vi "OSF Template.vi"(8 "error in":errorcluster, 9 "Proposal Data":T1, 10 "Token":string, 11 "OSF API URL":string="https://api.osf.io/v2/") -> (0 "error out":errorcluster)   [LabVIEW 2020]
uses:
  Utilities/iCalendar/Extract iCalendar String.ctl
  <vilib>/httpClient/LabVIEWHTTPClient.lvlib
  <vilib>/JDP Science/JSONtext/JSONtext.lvlib
panel:
  in  "Path to item":string="home1"
  in  "content":string
  in  "ID":string
  out "Display Text 2":string
  out "Display Text":string
  in  "Act":bool=TRUE
  in  "Responce body":string
  in  "Parse from":enum16{"Proposal HTML:", "Proposal cluster"}(ring)=enum."Proposal cluster"
  out "reply":string
  out "headers":string
  in  "Proposal document":path=path "C:/Users/l121767/Dropbox/Projects/FAIR/Project files/Proposal/National High Magnetic Field Laboratory - Users Program.html"
  out "resulting string":string
  out "body":string
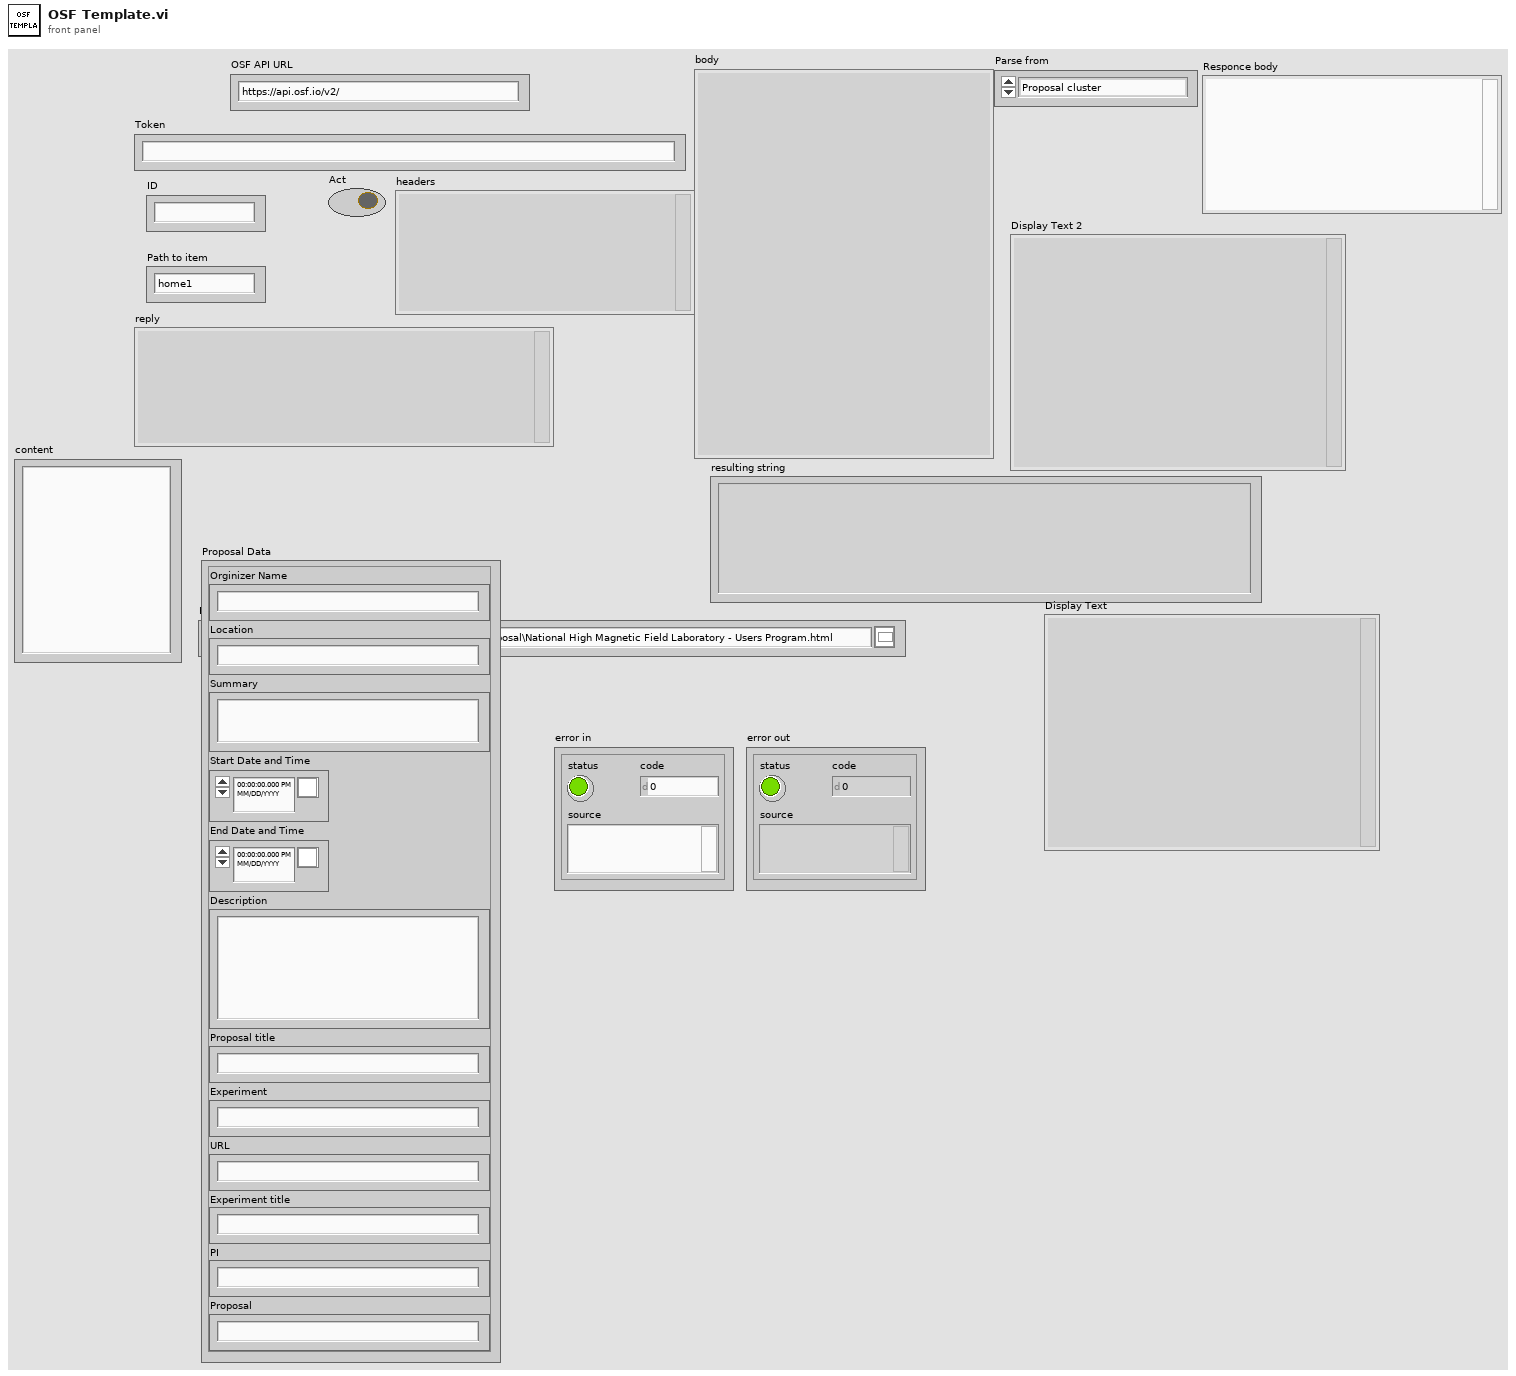
[diagram p1: front panel]
types:
  T1 = typedef "Extract iCalendar String.ctl" = cluster{"Orginizer Name":string, "Location":string, "Summary":string, "Start Date and Time":timestamp, "End Date and Time":timestamp, "Description":string, "Proposal title":string, "Experiment":string, "URL":string, "Experiment title":string, "PI":string, "Proposal":string}
  T2 = typedef "LabVIEWHTTPClient.lvlib/ClientHandle.ctl" = refnum<k1>
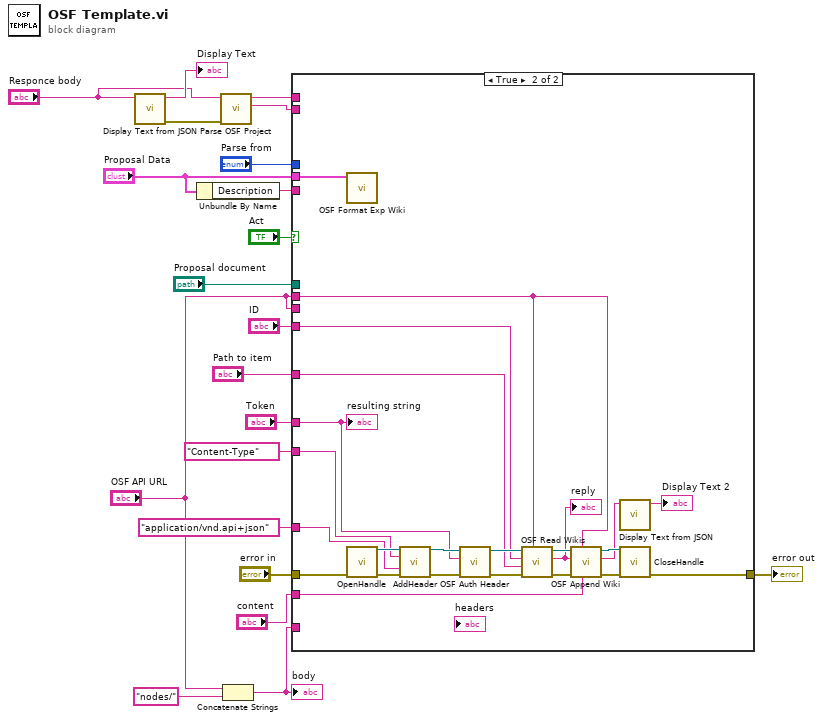
[diagram p0: block diagram]
diagram:
  n1 = call <vilib>:"Display Text from JSON.vi"("Input JSON"="Responce body") -> ("error out"=w8:errorcluster, "Display Text"=→"Display Text":string)  [unwired: 8 in, 1 out]
  n2 = Unbundle By Name("Proposal Data") -> ("Description"=w11:string)
  n3 = call "Parse OSF Project.vi"("error in"=w8, "Project JSON"="Responce body") -> ("Wiki href"=w6:string, "Project ID"=w5:string)  [unwired: 7 in, 1 out]
  n4 = Concatenate Strings("OSF API URL", "nodes/") -> (w16:string)
  "body" <- w16
  n5 = case shown="True" "Act" {
    tunnel: "Token" -> [_ w35]
    tunnel: "Content-Type" ("header") -> [_ w43]
    tunnel: "application/vnd.api+json" ("value") -> [_ w42]
    tunnel: "Proposal document" -> [_ _]
    tunnel: w16 -> [_ _]
    tunnel: "Parse from" -> [_ _]
    tunnel: "error in" -> [w22 w41]
    tunnel: [w22 w40] -> w13
    tunnel: "OSF API URL" -> [_ _]
    tunnel: "Proposal Data" -> [_ w38]
    tunnel: w11 -> [_ _]
    tunnel: w6 -> [_ _]
    tunnel: w5 -> [_ _]
    tunnel: "OSF API URL" -> [_ w25]
    tunnel: "ID" -> [_ w32]
    tunnel: "Path to item" -> [_ w31]
    tunnel: "content" -> [_ w23]
    frame False {
    }
    frame True {
      n6 = call "OSF Format Exp Wiki.vi"("Proposal Data"=w38) -> ()  [unwired: 9 in, 2 out]
      n7 = call <vilib>:"OpenHandle.vi"("error in (no error)"=w41) -> ("client handle out"=w45:T2, "error out"=w44:errorcluster)  [unwired: 13 in]
      n8 = call <vilib>:"AddHeader.vi"("client handle"=w45, "header"=w43, "value"=w42, "error in (no error)"=w44) -> ("client handle out"=w37:T2, "error out"=w34:errorcluster)  [unwired: 10 in]
      n9 = call "OSF Auth Header.vi"("error in"=w34, "Token"=w35, "client handle"=w37) -> ("error out"=w33:errorcluster, "client handle out"=w36:T2)  [unwired: 7 in]
      n10 = call "OSF Read Wikis.vi"("OSF API URL"=w25, "error in"=w33, "$Path or Item Name"=w31, "node"=w32, "client handle"=w36) -> ("error out"=w27:errorcluster, "Wiki ID"=w28:string, "client handle out"=w30:T2)  [unwired: 2 in, 2 out]
      "reply" <- w28
      n11 = call "OSF Append Wiki.vi"("content"=w23, "OSF API URL"=w25, "error in"=w27, "Wiki  ID"=w28, "client handle"=w30) -> ("error out"=w26:errorcluster, "Responce body"=w24:string, "client handle out"=w29:T2)  [unwired: 4 in]
      n12 = call <vilib>:"Display Text from JSON.vi"("Input JSON"=w24) -> ("Display Text"=→"Display Text 2":string)  [unwired: 8 in, 2 out]
      n13 = call <vilib>:"CloseHandle.vi"("client handle"=w29, "error in (no error)"=w26) -> ("error out"=w40:errorcluster)  [unwired: 13 in]
      "resulting string" <- w35
    }
  }
  "error out" <- w13
